vi "Write Action Type.vi"(8 "error in (no error)":errorcluster, 10 "Build Step":T1, 11 "Project Action in":refnum<class "Project Action.lvclass">) -> (0 "error out":errorcluster, 3 "Project Action out":refnum<class "Project Action.lvclass">)   [LabVIEW 2020, in "ProjectBuilder.lvlib" / "Project Action.lvclass"]
uses:
  Project Action.lvclass
  Sub/Private/Ctl/Ctl_Build Steps.ctl
  Project Action.lvclass/Project Action.ctl
  ProjectBuilder.lvlib
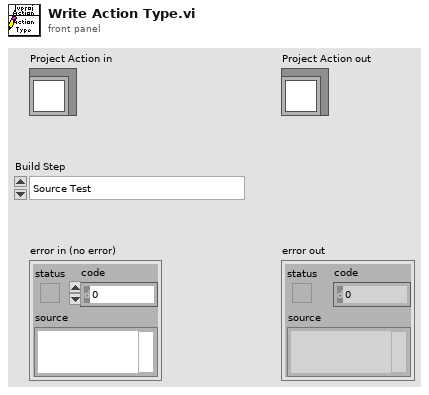
[diagram p1: front panel]
types:
  T1 = typedef "ProjectBuilder.lvlib/Ctl_Build Steps.ctl" = enum16{"Source Test", "Build", "Post-Build Test", "Deploy", "Report"}
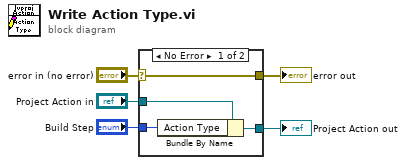
[diagram p0: block diagram]
diagram:
  n1 = case shown="No Error" "error in (no error)" {
    selector: "error in (no error)" -> [w9 w10]
    tunnel: [w9 w10] -> w4
    tunnel: [w7 w11] -> w2
    tunnel: "Project Action in" -> [w8 w11]
    tunnel: "Build Step" -> [w6 _]
    frame No Error {
      n2 = Bundle By Name(cluster=w8, "Action Type"=w6) -> (w7:refnum<class "Project Action.lvclass">)
    }
    frame Error {
    }
  }
  "error out" <- w4
  "Project Action out" <- w2
